vi "Start Receive Data.vi"(8 "error in (no error)":errorcluster, 11 "Tovey9150 in":refnum<class "Tovey 9150.lvclass">) -> (0 "error out":errorcluster, 3 "Tovey9150 out":refnum<class "Tovey 9150.lvclass">)   [LabVIEW 2015, in "Tovey 9150.lvclass"]
uses:
  Tovey 9150.lvclass
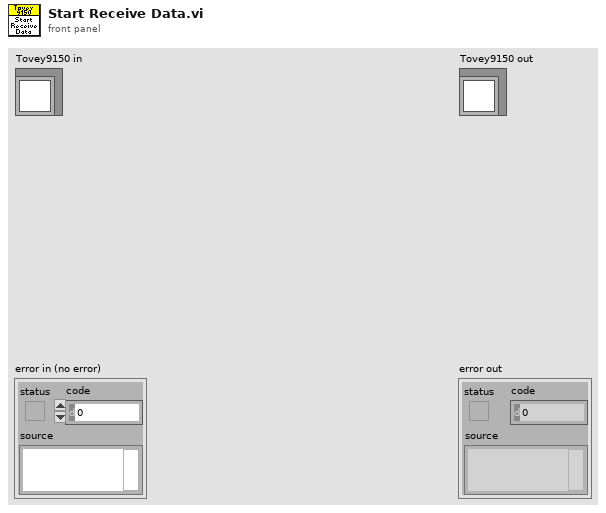
[diagram p1: front panel]
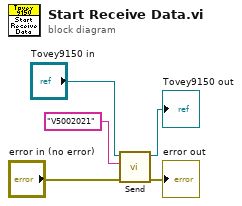
[diagram p0: block diagram]
diagram:
  n1 = call "Send.vi"("error in (no error)"="error in (no error)", "Message"="V5002021", "Tovey9150 in"="Tovey9150 in") -> ("error out"=→"error out":errorcluster, "Tovey9150 out"=→"Tovey9150 out":refnum<class "Tovey 9150.lvclass">)  [unwired: 7 in]
